vi "Find Resonances Interactive.vi"(8 "Error In":errorcluster) -> (0 "Error Out":errorcluster)   [LabVIEW 2016]
uses:
  Measure_extentions/Post-Processors/Line Detector/Line Detector Configuration.ctl
  <vilib>/Analysis/3filter.llb/Filter Passband Type.ctl
  <vilib>/Analysis/3filter.llb/Bessel Filter (CDB).vi
  Smooth Background CDBL.vi
  <vilib>/Analysis/NI_AALPro.lvlib
  <vilib>/Analysis/NI_AAL_SigProc.lvlib
  <vilib>/Analysis/NI_AALBase.lvlib
panel:
  in  "Low pass distortion":dbl
  out "XY Graph 6":cluster{dbl[], dbl[]}[](graph)
  in  "User configuration":T1={"Peak width"=30.0} {"Peak width" format="%#_6pHz"}
  in  "Signal channel":string="Signal"
  in  "Frequency channel":string="Frequency"
  in  "group name in":string="p"
  in  "HP F":dbl=0.1 format="%#_6p"
  in  "LP  F":dbl=0.001 format="%#_6p"
  in  "Fit?":bool
  in  "Complex":bool
  in  "Deviations":dbl=1.0
  out "variance":dbl format="%.2p"
  out "standard deviation":dbl format="%.2p"
  out "Peak F":dbl format="%#_6pHz"
  in  "Points around peak":i32=100
  in  "Peak number":i32
  out "XY Graph 5":cluster{"Array":dbl[], "Array":dbl[]}[](graph)
  out "width":i32=100 min=3
  out "XY Graph 4":cluster{"Y":dbl[], dbl[]}(graph)
  out "XY Graph 3":cluster{"Y":dbl[], "Y":dbl[]}[](graph)
  out "XY Graph 2":cluster{"Y":dbl[], dbl[]}[](graph)
  out "XY Graph":cluster{"Y":dbl[], "Unwrapped Phase":dbl[]}[](graph)
  in  "File Path Control":path=path "C:/Data/Spectra for Fedor/Ok spectra/300.00000K_175_555_2.10000V_0.00000T_May20-2015__09-37-18_001_052015.tdms"
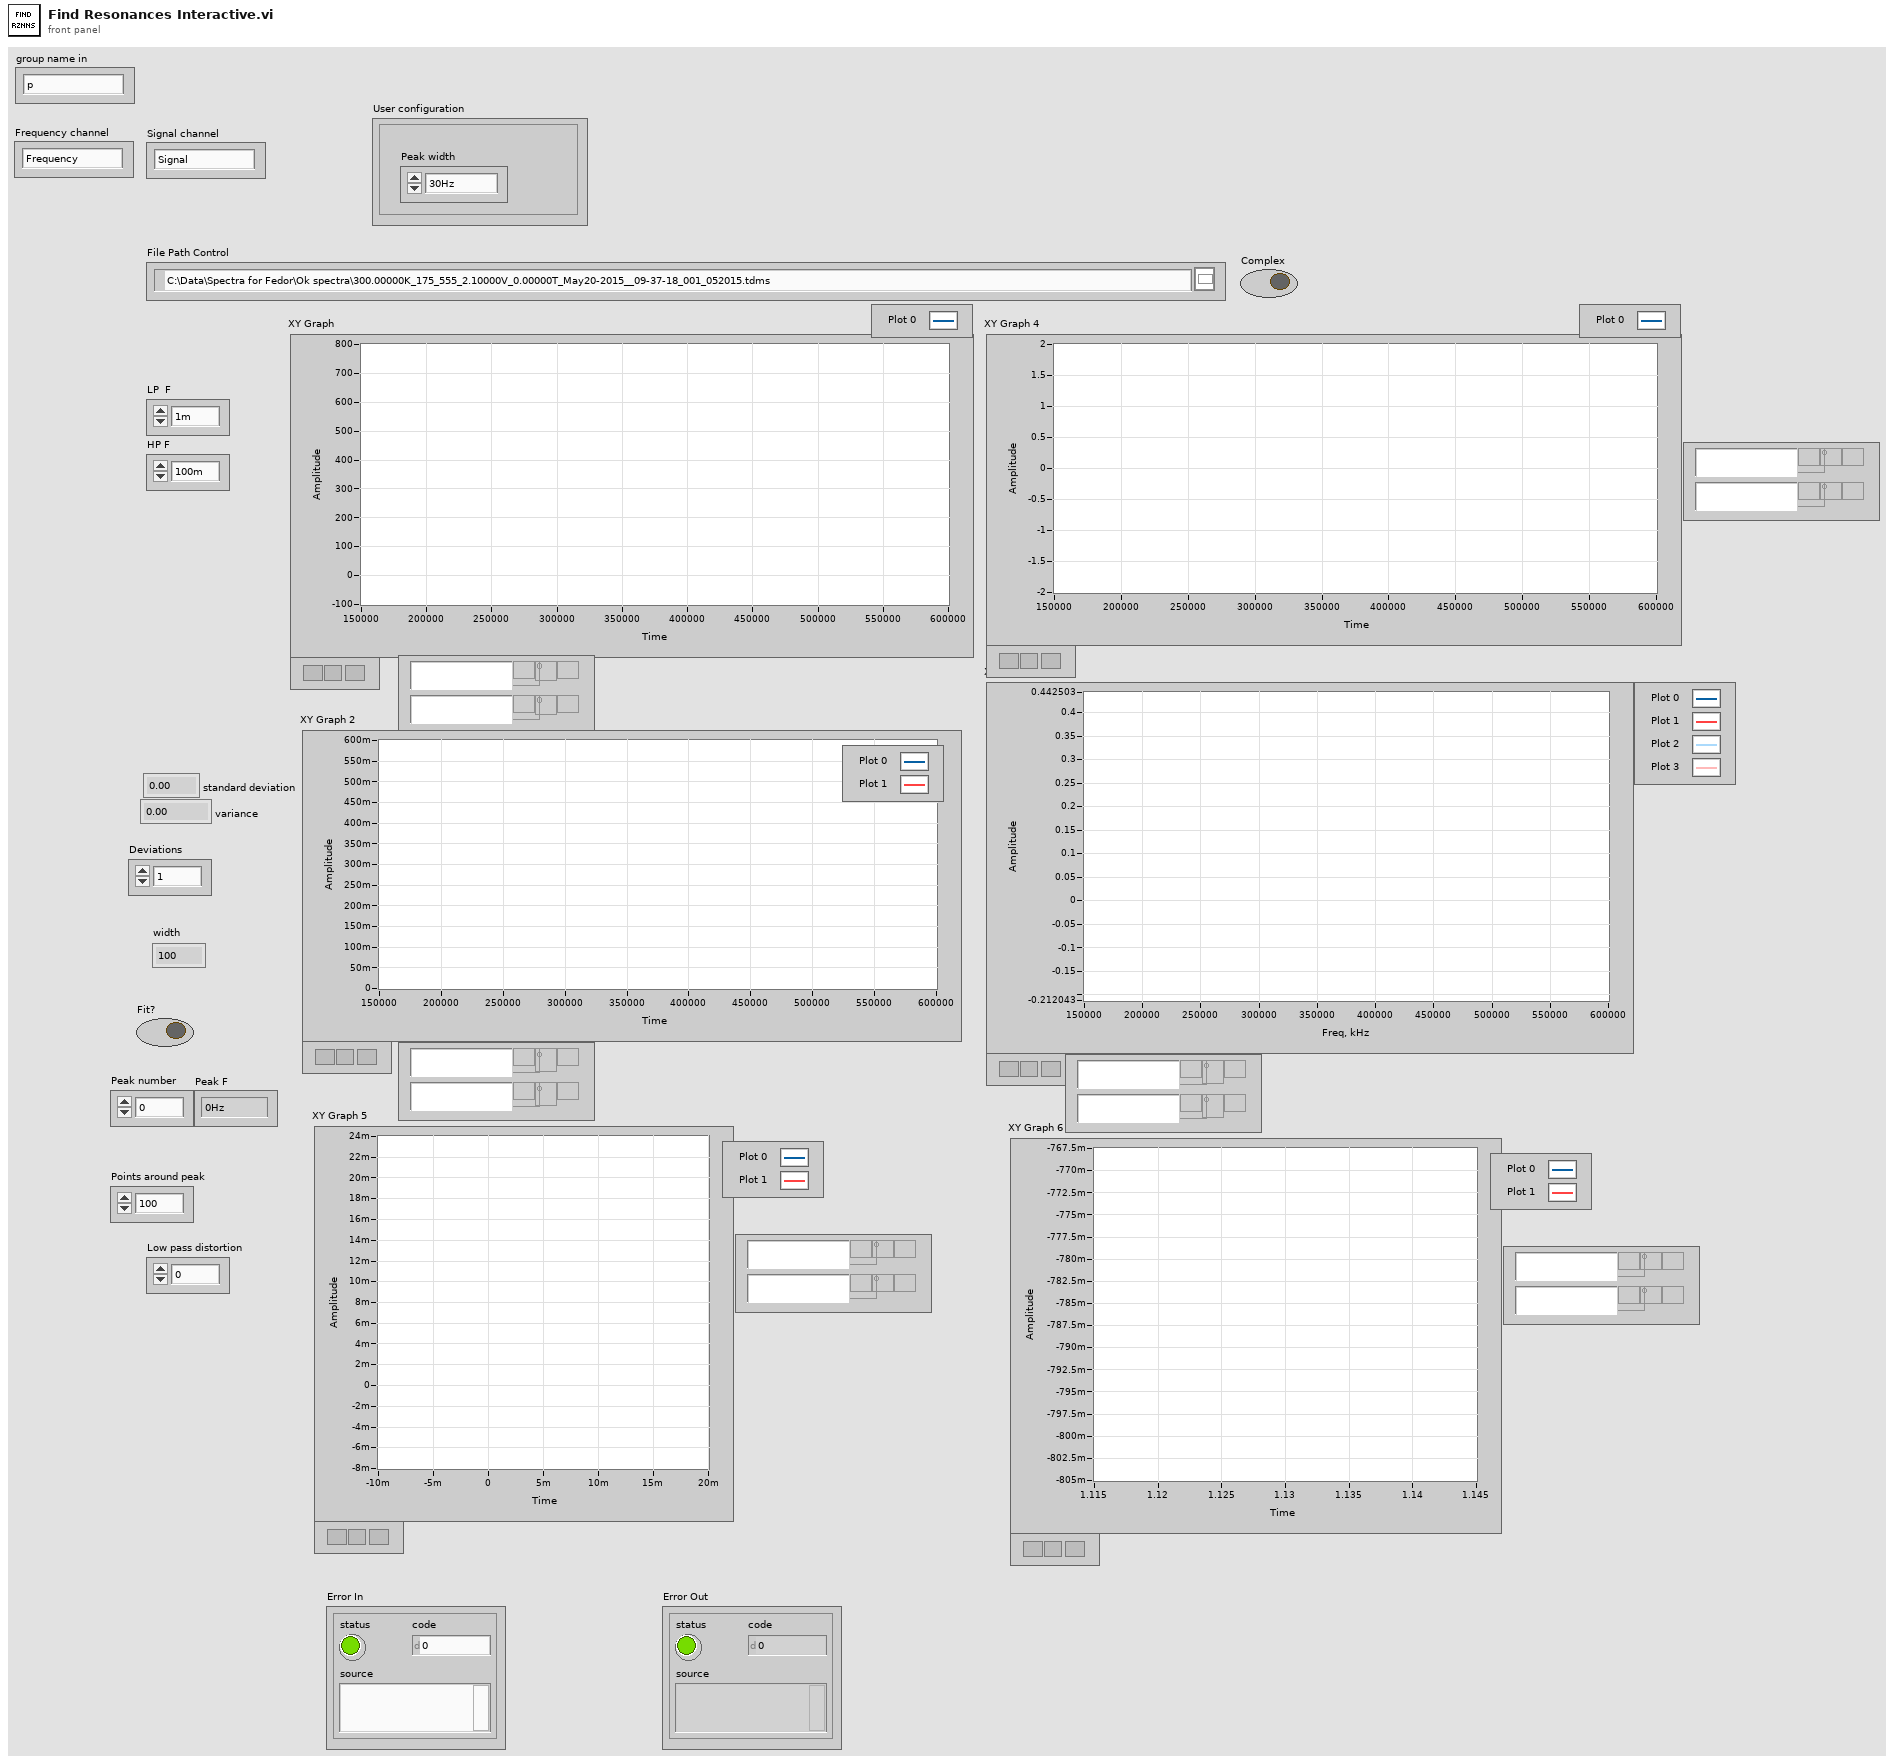
[diagram p1: front panel]
types:
  T1 = typedef "Line Detector Configuration.ctl" = cluster{"Peak width":dbl}
  T2 = enum16{"open", "open or create", "create or replace", "create", "open (read-only)"}
  T3 = typedef "NI_AALBase.lvlib/Filter Passband Type.ctl" = enum32{"Lowpass", "Highpass", "Bandpass", "Bandstop"}
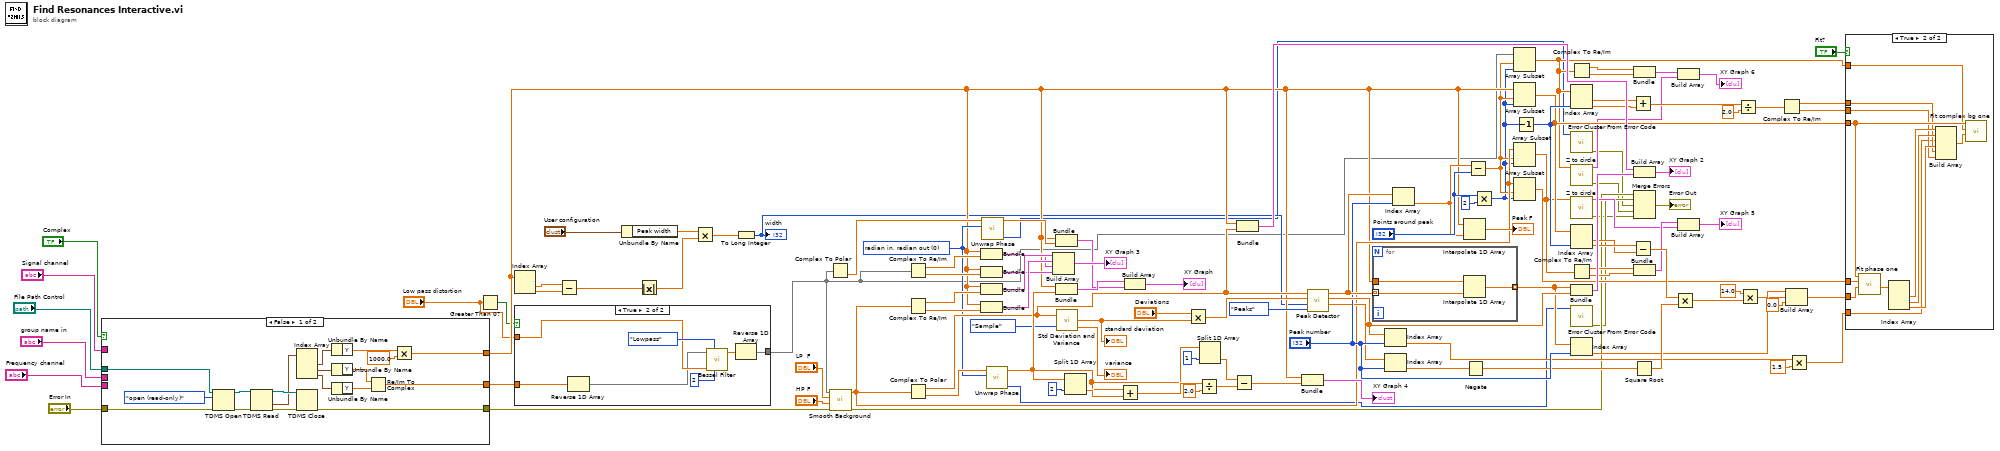
[diagram p0: block diagram]
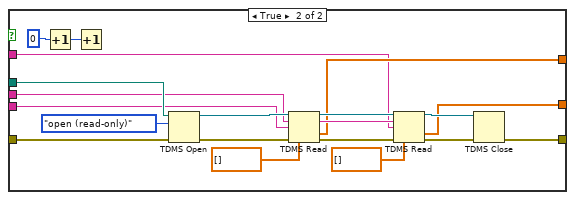
[diagram p4: hidden frame]
diagram:
  w78 = 0 items=["radian in, radian out", "radian in, degree out", "degree in, degree out", "degree in, radian out"] ("phase unit")
  n1 = case shown="False" "Complex" {
    tunnel: "File Path Control" -> [w134 w154]
    tunnel: [w118 w138] -> w36
    tunnel: "group name in" -> [_ w143]
    tunnel: "Frequency channel" -> [_ w142]
    tunnel: [w121 w139] -> w10
    tunnel: "Signal channel" -> [_ w137]
    tunnel: "Error In" -> [w120 w136]
    tunnel: [w119 w135] -> w37
    frame False {
      n2 = TDMS Open(8:w120, 10:T2."open (read-only)" ("operation (0:open)"), 11:w134) -> (0:w131:errorcluster, 3:w132:refnum<k34>)  [unwired: 4 in]
      n3 = TDMS Read(0:w132, 11:w131) -> (4:w130:refnum<k34>, 10:w128:waveform(dbl)[], 15:w129:errorcluster)  [unwired: 6 in, 3 out]
      n4 = Index Array(array=w128) -> (element #1=w127:waveform(dbl), element #2=w125:waveform(dbl), element #3=w126:waveform(dbl))  [unwired: 3 in]
      n5 = TDMS Close(8:w129, 11:w130) -> (0:w119:errorcluster)  [unwired: 1 out]
      n6 = Unbundle By Name(w127) -> ("Y"=w124:dbl[])
      n7 = Unbundle By Name(w125) -> ("Y"=w123:dbl[])
      n8 = Unbundle By Name(w126) -> ("Y"=w122:dbl[])
      n9 = Re/Im To Complex(1:w122, 2:w123) -> (0:w121:cdb[])
      n10 = Multiply(x=w124, y=1000.0) -> (x*y=w118:dbl[])
    }
    frame True {
      n11 = Increment(x=0 ("index")) -> (x+1=w148:i32)
      n12 = Increment(x=w148) -> ()  [unwired: 1 out]
      n13 = TDMS Open(8:w136, 10:T2."open (read-only)" ("operation (0:open)"), 11:w154) -> (0:w151:errorcluster, 3:w152:refnum<k34>)  [unwired: 4 in]
      n14 = TDMS Read(0:w152, 5:w143, 7:w142, 11:w151, 12:dbl[] []) -> (4:w146:refnum<k34>, 6:w144:string, 10:w138:dbl[], 15:w150:errorcluster)  [unwired: 3 in, 2 out]
      n15 = TDMS Read(0:w146, 5:w144, 7:w137, 11:w150, 12:cdb[] []) -> (4:w145:refnum<k34>, 10:w139:cdb[], 15:w147:errorcluster)  [unwired: 3 in, 3 out]
      n16 = TDMS Close(8:w147, 11:w145) -> (0:w135:errorcluster)  [unwired: 1 out]
    }
  }
  n17 = Greater Than 0?(x="Low pass distortion") -> (x > 0?=w12:bool)
  n18 = Index Array(array=w36) -> (element #1=w35:dbl, element #2=w34:dbl)  [unwired: 2 in]
  n19 = case shown="True" w12 {
    tunnel: w10 -> [w155 w162]
    tunnel: [w155 w156] -> w9
    tunnel: "Low pass distortion" -> [_ w159]
    frame False {
    }
    frame True {
      n20 = Reverse 1D Array(array=w162) -> (reversed array=w157:cdb[])
      n21 = call-poly <vilib>:"Bessel Filter.vi"("order"=2, "filter type"=Filter_Passband_Type."Lowpass", "low cutoff freq: fl"=w159, "X"=w157) -> ("Filtered X"=w161:cdb[])  [unwired: 4 in, 1 out]
      n22 = Reverse 1D Array(array=w161) -> (reversed array=w156:cdb[])
    }
  }
  n23 = Subtract(x=w35, y=w34) -> (x-y=w33:dbl)
  n24 = Unbundle By Name("User configuration") -> ("Peak width"=w31:dbl)
  n25 = Absolute Value(x=w33) -> (abs(x)=w30:dbl)
  n26 = Multiply(x=w31, y=w30) -> (x*y=w29:dbl)
  n27 = To Long Integer(number=w29) -> (32bit integer=w28:i32)
  "width" <- w28
  n28 = Complex To Polar(r * e^(i*theta)=w9) -> (theta=w77:dbl[])  [unwired: 1 out]
  n29 = call-poly "Smooth Background.vi"("Error In"=w37, "HP F"="HP F", "LP  F"="LP  F", "Data"=w9) -> ("Error Out"=w8:errorcluster, "Data out"=w48:cdb[])  [unwired: 6 in]
  n30 = Complex To Re/Im(x + iy=w9) -> (x=w88:dbl[], y=w89:dbl[])
  n31 = Complex To Re/Im(x + iy=w48) -> (x=w100:dbl[], y=w99:dbl[])
  n32 = Complex To Polar(r * e^(i*theta)=w48) -> (r=w85:dbl[], theta=w106:dbl[])
  n33 = Bundle(w36, w88) -> (w87:cluster{dbl[], dbl[]})  [unwired: 1 in]
  n34 = Bundle(w36, w89) -> (w86:cluster{dbl[], dbl[]})  [unwired: 1 in]
  n35 = Bundle(w36, w100) -> (w114:cluster{dbl[], dbl[]})  [unwired: 1 in]
  n36 = Bundle(w36, w99) -> (w113:cluster{dbl[], dbl[]})  [unwired: 1 in]
  n37 = call <vilib>:"Unwrap Phase.vi"("phase unit"=w78, "Phase"=w77) -> ("error"=w6:i32, "Unwrapped Phase"=w76:dbl[])  [unwired: 8 in]
  n38 = call <vilib>:"Unwrap Phase.vi"("phase unit"=w78, "Phase"=w106) -> ("error"=w7:i32, "Unwrapped Phase"=w101:dbl[])  [unwired: 8 in]
  n39 = Build Array(w114, w113, w87, w86) -> (→"XY Graph 3":cluster{dbl[], dbl[]}[])
  n40 = Bundle(w36, "Unwrapped Phase"=w76) -> (w74:cluster{dbl[], "Unwrapped Phase":dbl[]})  [unwired: 1 in]
  n41 = Bundle(w36, "Unwrapped Phase"=w101) -> (w115:cluster{dbl[], "Unwrapped Phase":dbl[]})  [unwired: 1 in]
  n42 = call <vilib>:"Std Deviation and Variance.vi"("X"=w85, "Weighting (Sample)"=enum16{"Sample", "Population"}."Sample") -> ("standard deviation"=w80:dbl, "variance"=→"variance":dbl)  [unwired: 1 out]
  "standard deviation" <- w80
  n43 = Split 1D Array(array=w101, index=2) -> (second subarray=w109:dbl[])  [unwired: 1 out]
  n44 = Add(x=w101, y=w109) -> (x+y=w108:dbl[])
  n45 = Build Array(w115, w74) -> (→"XY Graph":cluster{dbl[], "Unwrapped Phase":dbl[]}[])
  n46 = Multiply(x="Deviations", y=w80) -> (x*y=w81:dbl)
  n47 = Divide(x=w108, y=2.0) -> (x/y=w105:dbl[])
  n48 = Split 1D Array(array=w101, index=1) -> (second subarray=w102:dbl[])  [unwired: 1 out]
  n49 = Subtract(x=w102, y=w105) -> (x-y=w104:dbl[])
  n50 = Bundle(w36, w85) -> (w98:cluster{dbl[], dbl[]})  [unwired: 1 in]
  n51 = Bundle(w36, w104) -> (→"XY Graph 4":cluster{dbl[], dbl[]})  [unwired: 1 in]
  n52 = call <vilib>:"Peak Detector.vi"("peaks/valleys"=enum32{"Peaks", "Valleys"}."Peaks", "width"=w28, "threshold"=w81, "X"=w85) -> ("2nd Derivatives"=w64:dbl[], "Amplitudes"=w71:dbl[], "Locations"=w66:dbl[])  [unwired: 3 in, 2 out]
  n53 = for {
    tunnel: w36 -> [w165]
    tunnel: w66 -> [w164] mode=indexing
    tunnel: [w163] -> w70 mode=indexing
    n54 = Interpolate 1D Array(1:w164, 2:w165) -> (0:w163:dbl)
  }
  n55 = Index Array(array=w71, index="Peak number") -> (element=w43:dbl)
  n56 = Index Array(array=w64, index="Peak number") -> (element=w63:dbl)
  n57 = Index Array(array=w66, index="Peak number") -> (element=w72:dbl)
  n58 = Interpolate 1D Array(1:w72, 2:w36) -> (0:→"Peak F":dbl)
  n59 = Negate(x=w63) -> (-x=w60:dbl)
  n60 = Subtract(x=w72, y="Points around peak") -> (x-y=w25:dbl)
  n61 = Multiply(x="Points around peak", y=2) -> (x*y=w24:i32)
  n62 = Array Subset(array=w9, index=w25, length=w24) -> (w18:cdb[])
  n63 = Array Subset(array=w36, index=w25, length=w24) -> (w23:dbl[])
  n64 = Array Subset(array=w48, index=w25, length=w24) -> (w16:cdb[])
  n65 = Array Subset(array=w48, index=w25, length=w24) -> (w49:cdb[])
  n66 = Decrement(x=w24) -> (x-1=w69:i32)
  n67 = Index Array(array=w18, index #2=w69) -> (element #1=w59:cdb, element #2=w58:cdb)  [unwired: 1 in]
  n68 = call <vilib>:"Error Cluster From Error Code.vi"("error code (0)"=w6) -> ("error out"=w3:errorcluster)  [unwired: 8 in]
  n69 = call "Z to circle.vi"("Z"=w18) -> ("Error Out"=w2:errorcluster, "plot"=w17:cluster{"Array":dbl[], "Array":dbl[]})  [unwired: 6 in, 3 out]
  n70 = call "Z to circle.vi"("Z"=w16) -> ("Error Out"=w1:errorcluster, "plot"=w14:cluster{"Array":dbl[], "Array":dbl[]})  [unwired: 6 in, 3 out]
  n71 = Index Array(array=w23, index #2=w69) -> (element #1=w67:dbl, element #2=w68:dbl)  [unwired: 1 in]
  n72 = Bundle(w70, "Amplitudes"=w71) -> (w95:cluster{dbl[], "Amplitudes":dbl[]})  [unwired: 1 in]
  n73 = call <vilib>:"Error Cluster From Error Code.vi"("error code (0)"=w7) -> ("error out"=w4:errorcluster)  [unwired: 8 in]
  n74 = Index Array(array=w70, index="Peak number") -> (element=w56:dbl)
  n75 = Complex To Re/Im(x + iy=w18) -> (x=w21:dbl[], y=w20:dbl[])
  n76 = Complex To Re/Im(x + iy=w16) -> (x=w92:dbl[], y=w91:dbl[])
  n77 = Add(x=w59, y=w58) -> (x+y=w57:cdb)
  n78 = Subtract(x=w68, y=w67) -> (x-y=w61:dbl)
  n79 = Square Root(x=w60) -> (sqrt(x)=w62:dbl)
  n80 = Bundle(w21, w20) -> (w22:cluster{dbl[], dbl[]})  [unwired: 1 in]
  n81 = Build Array(w98, w95) -> (→"XY Graph 2":cluster{dbl[], "Amplitudes":dbl[]}[])
  n82 = Merge Errors(w8, w4, w3, w2, w1) -> (→"Error Out":errorcluster)
  n83 = Bundle(w92, w91) -> (w15:cluster{dbl[], dbl[]})  [unwired: 1 in]
  n84 = Multiply(x=w61, y=w62) -> (x*y=w55:dbl)
  n85 = Build Array(w22, w17) -> (→"XY Graph 6":cluster{"Array":dbl[], "Array":dbl[]}[])
  n86 = Build Array(w15, w14) -> (→"XY Graph 5":cluster{"Array":dbl[], "Array":dbl[]}[])
  n87 = Divide(x=w57, y=2.0) -> (x/y=w52:cdb)
  n88 = Multiply(x=14.0, y=w55) -> (x*y=w27:dbl)
  n89 = Complex To Re/Im(x + iy=w52) -> (x=w51:dbl, y=w50:dbl)
  n90 = Build Array(w56, w27, 0.0 ("element")) -> (w53:dbl[])
  n91 = Multiply(x=w43, y=1.5) -> (x*y=w42:dbl)
  n92 = case shown="True" "Fit?" {
    tunnel: w18 -> [_ w176]
    tunnel: w23 -> [_ w177]
    tunnel: w53 -> [_ w175]
    tunnel: w42 -> [_ w167]
    tunnel: w51 -> [_ w170]
    tunnel: w50 -> [_ w169]
    tunnel: w49 -> [_ w166]
    frame False {
    }
    frame True {
      n93 = call "Fit phase one.vi"("Initial parameters"=w175, "Z"=w166, "X"=w177) -> ("best fit parameters"=w174:dbl[])  [unwired: 7 in, 1 out]
      n94 = Index Array(array=w174) -> (element #1=w173:dbl, element #2=w172:dbl, element #3=w171:dbl)  [unwired: 3 in]
      n95 = Build Array(w173, w172, w167, w171, w170, w169) -> (w168:dbl[])
      n96 = call "Fit complex bg one.vi"("Initial parameters"=w168, "Z"=w176, "X"=w177) -> ()  [unwired: 8 in, 1 out]
    }
  }
